vi "NISE.local.Initialize (Physical Channel).vi"(0 "physical channels":refnum<k21>, 7 "reservation access (Read/Write)":i32(ring)=3 items=["None"=0, "Read Only"=1, "Read/Write"=3], 9 "reservation group":string, 11 "error in (no error)":errorcluster, 12 "connect timeout (60 sec)":dbl=60.0) -> (4 "SLSC Local out":refnum<class "SLSC Interface.lvclass">, 15 "error out":errorcluster)   [LabVIEW 2016, in "SLSC Interface.lvclass"]
uses:
  SLSC Interface Class/SLSC Interface.lvclass
  <vilib>/SLSC/Initialize Session with Phys Chans.vi
  SLSC Interface Class/NISE.Write session.vi
  <vilib>/SLSC/SLSC.lvlib
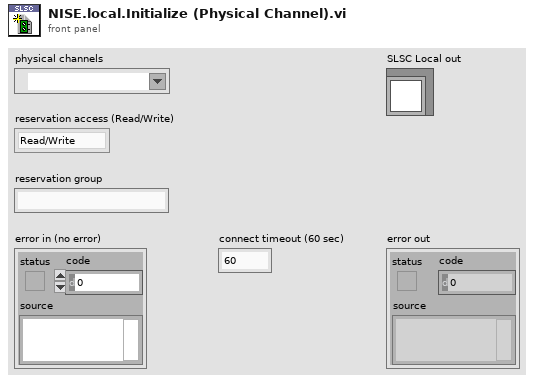
[diagram p1: front panel]
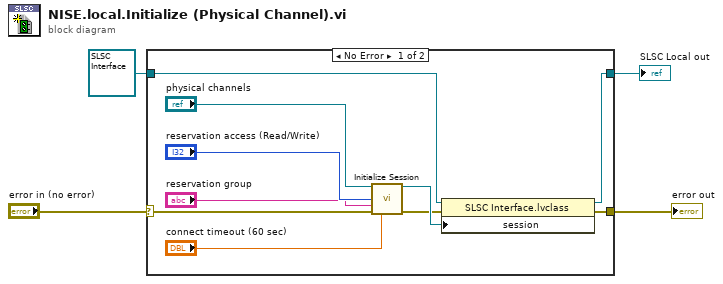
[diagram p0: block diagram]
diagram:
  n1 = case shown="No Error" "error in (no error)" {
    selector: "error in (no error)" -> [w14 w16]
    tunnel: [w5 w16] -> w3
    tunnel: [w7 w15] -> w2
    tunnel: refnum<class "SLSC Interface.lvclass"> refnum ("SLSC Interfaces.lvlib:SLSC Interface.lvclass") -> [w9 w15]
    frame No Error {
      n2 = call-poly <vilib>:"Initialize Session.vi"("physical channels"="physical channels", "reservation access (Read/Write)"="reservation access (Read/Write)", "reservation group"="reservation group", "error in (no error)"=w14, "connect timeout (60 sec)"="connect timeout (60 sec)") -> ("session out"=w8:refnum<k21>, "error out"=w6:errorcluster)  [unwired: 9 in]
      n3 = property class="SLSC Interface.lvclass"(reference=w9, error in=w6, "session"=w8) -> (reference out=w7:refnum<class "SLSC Interface.lvclass">, error out=w5:errorcluster)
    }
    frame Error {
    }
  }
  "error out" <- w3
  "SLSC Local out" <- w2
